vi "Sub Initialize.vi"(6 "Controller name":string, 8 "error in (no error)":errorcluster, 11 "Instrument Recorder in":refnum<class "Combined Measurement.lvclass">) -> (0 "error out":errorcluster, 2 "Initialize Result":refnum<class "Acquired Result.lvclass">, 3 "Instrument Recorder out":refnum<class "Combined Measurement.lvclass">)   [LabVIEW 2021, in "Combined Measurement.lvclass"]
uses:
  Combined Measurement.lvclass
  C:/Program Files/National Instruments/LabVIEW 2021/vi.lib/ActorFramework/Actor/Actor.lvclass
  NHMFL_Core/Libraries/Instruments/Results/Acquired Result/Acquired Result.lvclass
  <vilib>/ActorFramework/Actor/Actor.lvclass/Actor.ctl
  <vilib>/ActorFramework/Message Enqueuer/Message Enqueuer.lvclass/Message Enqueuer.ctl
  <vilib>/ActorFramework/Message Enqueuer/Init from Existing Queue.vi
  Measurements/Response Synchronizer/Response Synchronizer.lvclass
  <vilib>/ActorFramework/Message Enqueuer/Message Enqueuer.lvclass
  Continuous Recorder Actor/Continuous Recorder Actor.lvclass
  <vilib>/ActorFramework/Actor/Actor.lvclass
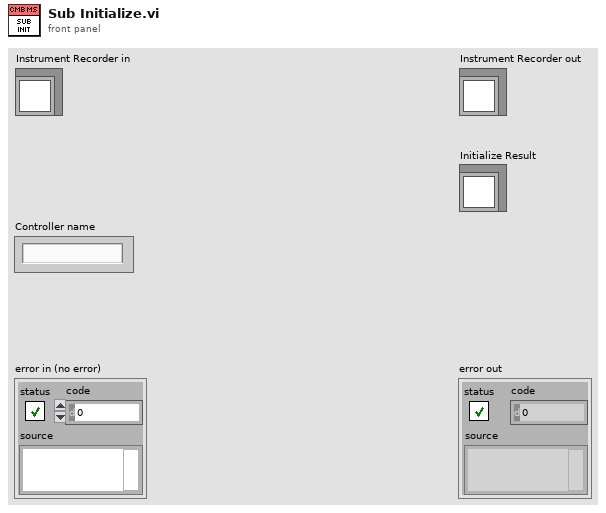
[diagram p1: front panel]
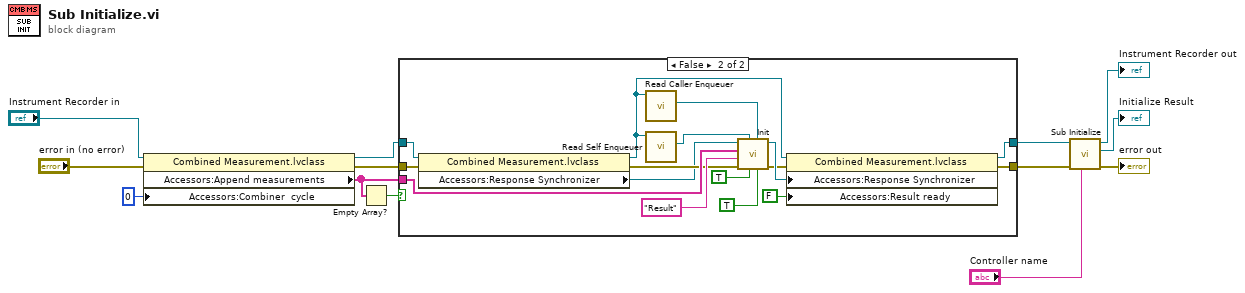
[diagram p0: block diagram]
diagram:
  n1 = property class="Combined Measurement.lvclass"(reference="Instrument Recorder in", error in="error in (no error)", "Accessors:Combiner  cycle"=0 ("Combiner  cycle")) -> (reference out=w7:refnum<class "Combined Measurement.lvclass">, error out=w5:errorcluster, "Accessors:Append measurements"=w6:string[])
  n2 = Empty Array?(array=w6) -> (empty?=w8:bool)
  n3 = case shown="False" w8 {
    tunnel: [w15 w20] -> w4
    tunnel: w5 -> [w14 w26]
    tunnel: [w14 w18] -> w2
    tunnel: w6 -> [_ w29]
    tunnel: w7 -> [w15 w24]
    frame True {
    }
    frame False {
      n4 = property class="Combined Measurement.lvclass"(reference=w24, error in=w26) -> (reference out=w21:refnum<class "Combined Measurement.lvclass">, error out=w25:errorcluster, "Accessors:Response Synchronizer"=w23:refnum<class "Response Synchronizer.lvclass">)
      n5 = call <vilib>:"Read Caller Enqueuer.vi"("Actor"=w21) -> ("Caller Enqueuer"=w28:refnum<class "Message Enqueuer.lvclass">)  [unwired: 10 in]
      n6 = call <vilib>:"Read Self Enqueuer.vi"("Actor"=w21) -> ("Self Enqueuer"=w27:refnum<class "Message Enqueuer.lvclass">)  [unwired: 10 in]
      n7 = call-dynamic "Init.vi"("Pre-preocess datasockets"=TRUE, "Caller Enqueuer"=w28, "Subscribe"=TRUE, "Self Enqueuer"=w27, "error in (no error)"=w25, "Topic"="Result", "Responder names"=w29, "Response Synchronizer in"=w23) -> ("error out"=w19:errorcluster, "Response Synchronizer out"=w22:refnum<class "Response Synchronizer.lvclass">)  [unwired: 2 in]
      n8 = property class="Combined Measurement.lvclass"(reference=w21, error in=w19, "Accessors:Response Synchronizer"=w22, "Accessors:Result ready"=FALSE ("Result ready")) -> (reference out=w20:refnum<class "Combined Measurement.lvclass">, error out=w18:errorcluster)
    }
  }
  n9 = call-parent "Sub Initialize.vi"("Controller name"="Controller name", "error in (no error)"=w2, "Instrument Recorder in"=w4) -> ("error out"=→"error out":errorcluster, "Initialize Result"=→"Initialize Result":refnum<class "Acquired Result.lvclass">, "Instrument Recorder out"=→"Instrument Recorder out":refnum<class "Combined Measurement.lvclass">)  [unwired: 6 in]
